vi "BonOMM-SAOMM.Test.vi"() -> ()   [LabVIEW 2011] (continued)
                        n1500 = case shown="False" w5027 {
                          frame False {
                            n1501 = One Button Dialog(message="ATTENTION!!\nLe télescope n'est pas en \nMODE ENTRAÎNEMENT SIDÉRAL.", button name ("OK")="OK" ("nom du bouton (\"OK\")")) -> ()  [unwired: 1 out]
                          }
                          frame True {
                          }
                        }
                      }
                    }
                  }
                }
                n1502 = case shown="True" w5001 {
                  frame False {
                  }
                  frame True {
                    n1503 = property on="GO" class="Bool (strict)"("Key Focus"=TRUE) -> ()  [unwired: 2 in, 2 out]
                  }
                }
              }
              event "SaveCoords": Value Change {
                n1504 = event-data() -> ()  [unwired: 1 in, 5 out]
                n1505 = flat-sequence {
                  tunnel: [w5039] -> w5035
                  tunnel: [w5038] -> w5034
                  tunnel: [w5037] -> w5033
                  tunnel: [w5036] -> w5032
                  tunnel: w5035 -> [w5045]
                  tunnel: w5034 -> [w5046]
                  tunnel: w5033 -> [w5047]
                  tunnel: w5032 -> [w5044]
                  frame #0 {
                    n1506 = local read "Epoch Tel"() -> (w5040:dbl)
                    n1507 = local read "DEC Tel"() -> (w5042:dbl)
                    n1508 = local read "RA Tel"() -> (w5041:dbl)
                    n1509 = local write "SaveCoords"(FALSE ("SaveCoords")) -> ()
                    n1510 = call "SaveCoords.vi"("Epoch Tel"=w5040, "DEC Tel"=w5042, "RA Tel"=w5041) -> ("Accepted?"=w5036:bool, "Epoch Out"=w5037:dbl, "DEC Out"=w5038:dbl, "RA Out"=w5039:dbl)  [unwired: 5 in]
                  }
                  frame #1 {
                    n1511 = case shown="True" w5044 {
                      tunnel: w5047 -> [_ w5051]
                      tunnel: w5046 -> [_ w5050]
                      tunnel: w5045 -> [_ w5049]
                      frame False {
                      }
                      frame True {
                        w5075 = "\t"
                        w5068 = "_"
                        w5062 = TRUE ("replace all? (F)")
                        w5061 = " "
                        w5060 = "0"
                        w5057 = i16 2 ("width (-)")
                        w5056 = i16 0 ("width (-)")
                        n1512 = call "time-sec-to-time-str-DEC.vi"("Numeric"=w5049) -> ("formatted-str"=w5072:string)
                        n1513 = call "time-sec-to-time-str-DEC.vi"("Numeric"=w5050) -> ("formatted-str"=w5073:string)
                        n1514 = Number To Fractional String(number=w5051, width (-)=i16 4, precision (6)=i16 2) -> (F-format string=w5074:string)  [unwired: 1 in]
                        n1515 = Get Date/Time String() -> (time string=w5071:string)  [unwired: 3 in, 1 out]
                        n1516 = local read "From library"() -> (w5052:bool)
                        n1517 = Concatenate Strings(w5071, w5075, w5072, w5075, w5073, w5075, w5074, "\r\n") -> (w5077:string)
                        n1518 = call "GetUTC.vi"() -> ("Day"=w5082:dbl, "Month"=w5081:dbl, "Year"=w5080:dbl)  [unwired: 6 out]
                        n1519 = case shown="True" w5052 {
                          tunnel: [FALSE FALSE] -> w5048
                          tunnel: w5072 -> [w5086 w5093]
                          tunnel: w5073 -> [w5085 w5094]
                          tunnel: w5074 -> [w5084 w5095]
                          tunnel: w5071 -> [w5083 w5092]
                          frame False {
                            w5088 = i16 0 items=["tel coords", "tel offset", "guidage"] ("options")
                            n1520 = local read "Obslib"() -> (w5089:string[][])
                            n1521 = Build Array(w5086, w5085, w5084, w5083) -> (w5090:string[])
                            n1522 = call "Coords to chart(new).vi"("DataLine"=w5090, "options"=w5088, "Tableau entrant"=w5089) -> ("historique"=w5091:string[][])
                            n1523 = local write "Obslib"(w5091) -> ()
                          }
                          frame True {
                            w5097 = i16 0 items=["tel coords", "tel offset", "guidage"] ("options")
                            n1524 = local read "Obslib"() -> (w5098:string[][])
                            n1525 = Build Array(w5093, w5094, w5095, w5092) -> (w5099:string[])
                            n1526 = call "Coords to chart(new).vi"("DataLine"=w5099, "options"=w5097, "Tableau entrant"=w5098) -> ("historique"=w5100:string[][])
                            n1527 = local write "Obslib"(w5100) -> ()
                          }
                        }
                        n1528 = Number To Fractional String(number=w5080, width (-)=i16 4, precision (6)=w5056) -> (F-format string=w5063:string)  [unwired: 1 in]
                        n1529 = Number To Fractional String(number=w5081, width (-)=w5057, precision (6)=w5056) -> (F-format string=w5058:string)  [unwired: 1 in]
                        n1530 = Number To Fractional String(number=w5082, width (-)=w5057, precision (6)=w5056) -> (F-format string=w5059:string)  [unwired: 1 in]
                        n1531 = Search and Replace String(replace all?=w5062, input string=w5058, search string=w5061, replace string=w5060) -> (result string=w5064:string)  [unwired: 4 in, 3 out]
                        n1532 = Search and Replace String(replace all?=w5062, input string=w5059, search string=w5061, replace string=w5060) -> (result string=w5065:string)  [unwired: 4 in, 3 out]
                        n1533 = local read "path_pointing"() -> (w5066:path)
                        n1534 = Concatenate Strings(w5063, w5068, w5064, w5068, w5065, ".pnt") -> (w5067:string)
                        n1535 = Build Path(base path=w5066, name or relative path=w5067) -> (appended path=w5070:path)
                        n1536 = local read "File I/O Error"() -> (w5079:errorcluster)
                        n1537 = Write to Text File(file (use dialog)=w5070, text=w5077, error in=w5079) -> (error out=w5078:errorcluster)  [unwired: 1 in, 2 out]
                        n1538 = local write "From library"(w5048) -> ()
                        n1539 = local write "File I/O Error"(w5078) -> ()
                      }
                    }
                  }
                }
              }
              event "NO RA clic-sim": Value Change; "N.O. A.D.": Mouse Down {
                n1540 = event-data() -> ()  [unwired: 1 in, 4 out]
                n1541 = local write "N.O. A.D."("") -> ()
                n1542 = local write "NO epoch"(2000.0 ("NO epoch")) -> ()
                "NO RA clic-sim" <- FALSE
              }
              event "N.O. Déc.": Mouse Down {
                n1543 = event-data() -> ()  [unwired: 1 in, 8 out]
                n1544 = local write "NO epoch"(2000.0 ("NO epoch")) -> ()
                n1545 = local write "N.O. Déc."("") -> ()
              }
              event "Zénith", "Écran", "Range": Value Change {
                n1546 = event-data() -> ()  [unwired: 1 in, 1 out]
                n1547 = local read "Mode Est"() -> (w5106:bool)
                n1548 = case shown="False" w5106 {
                  selector: w5106 -> [_ w5319]
                  frame False {
                    # "Track ON ou OFF"
                    n1549 = local read "STATL"() -> (w5111:bool[])
                    n1550 = Index Array(array=w5111, index=2 ("Index")) -> (element=w5110:bool)
                    n1551 = case shown="False" w5110 {
                      tunnel: "Range" -> [w5116 _]
                      tunnel: "Zénith" -> [w5115 _]
                      tunnel: "Écran" -> [w5114 _]
                      frame False {
                        w5113 = FALSE
                        w5119 = string[] ["RANGEMENT", "ZÉNITH", "ÉCRAN"]
                        w5124 = 0
                        n1552 = local read "TCS VRN"() -> (w5123:refnum<visa-resource-name>)
                        n1553 = control-ref of="TERMINAL"() -> (w5121:refnum<vi>)
                        n1554 = control-ref of="Indicateur d'état"() -> (w5122:refnum<vi>)
                        n1555 = Select(t=1, s=w5116, f=w5124) -> (s? t:f=w5132:i32)
                        n1556 = Select(t=2, s=w5115, f=w5124) -> (s? t:f=w5130:i32)
                        n1557 = Select(t=3, s=w5114, f=w5124) -> (s? t:f=w5131:i32)
                        n1558 = Compound Arithmetic op=ADD(w5132, w5130, w5131) -> (w5129:i32)
                        n1559 = local write "Zénith"(w5113) -> ()
                        n1560 = local write "Écran"(w5113) -> ()
                        n1561 = local write "Range"(w5113) -> ()
                        n1562 = Decrement(x=w5129) -> (x-1=w5120:i32)
                        n1563 = Index String Array(1:w5120, 2:w5119, 3:"Le télescope va se déplacer\nvers la position ") -> (0:w5128:string)
                        n1564 = Two Button Dialog(message=w5128, 1:"Annulez" ("Nom du bouton F (\"Annuler\")"), 2:"OK" ("Nom du bouton V (\"OK\")")) -> (T button?=w5136:bool)
                        n1565 = Index String Array(1:w5120, 2:w5119, 3:"Commande de déplacement : " ("string (\"\")")) -> (0:w5117:string)
                        n1566 = call "TERMINAL.vi"("Indicateur Refnum"=w5122, "Terminal Refnum"=w5121, "Indicateur d'état"=w5117) -> ()
                        n1567 = case shown="True" w5136 {
                          selector: w5136 -> [w5137 _]
                          tunnel: w5120 -> [_ w5141]
                          tunnel: w5116 -> [_ w5140]
                          tunnel: w5119 -> [_ w5139]
                          tunnel: w5123 -> [_ w5138]
                          frame False {
                            n1568 = local write "Zénith"(w5137) -> ()
                            n1569 = local write "Écran"(w5137) -> ()
                            n1570 = local write "Range"(w5137) -> ()
                          }
                          frame True {
                            n1571 = stacked-sequence {
                              seq-local: [w5143 _ _] -> [_ _ w5311]
                              tunnel: w5141 -> [w5144 w5172 _]
                              tunnel: w5140 -> [_ w5179 _]
                              tunnel: w5139 -> [_ w5178 _]
                              tunnel: w5138 -> [w5142 w5177 _]
                              frame #0 {
                                n1572 = disable-structure shown="Disabled" {
                                disable-tunnel: [w5146 _] -> w5143
                                disable-tunnel: w5142 -> [w5145 _]
                                frame Disabled {
                                n1573 = flat-sequence {
                                tunnel: [w5148] -> w5146
                                tunnel: w5145 -> [w5152]
                                tunnel: [w5150] -> w5147
                                tunnel: w5147 -> [w5155]
                                frame #0 {
                                n1574 = local read "Epoch Tel"() -> (w5149:dbl)
                                n1575 = Build Array(w5149) -> (w5148:dbl[])
                                }
                                frame #1 {
                                n1576 = local read "AnnéeRL"() -> (w5150:dbl)
                                n1577 = control-ref of="TCS actif"() -> (w5151:refnum<vi>)
                                n1578 = Build Array(w5150) -> (w5154:dbl[])
                                n1579 = call "EXCOM-CMD.vi"("VRN IN"=w5152, "Bool Refnum"=w5151, "Commande #"=22, "Args"=w5154) -> ()  [unwired: 9 in, 3 out]
                                }
                                frame #2 {
                                n1580 = while {
                                tunnel: [w5158] -> _
                                tunnel: w5155 -> [w5156]
                                i -> [w5165]
                                stop <- w5162 stop-if-true
                                # "Environ 1 jour ..."
                                n1581 = local read "Epoch Tel"() -> (w5161:dbl)
                                n1582 = Subtract(x=w5161, y=w5156) -> (x-y=w5160:dbl)
                                n1583 = Absolute Value(x=w5160) -> (abs(x)=w5159:dbl)
                                n1584 = Less Or Equal?(x=w5159, y=0.002) -> (x <= y?=w5158:bool)
                                n1585 = call "Max-iteration.vi"("i max"=500, "i act"=w5165, "Valeur entrante"=w5158) -> ("break ?"=w5162:bool)
                                n1586 = Wait (ms)(milliseconds to wait=u32 10) -> ()  [unwired: 1 out]
                                }
                                }
                                }
                                }
                                frame Enabled {
                                }
                                }
                                n1587 = disable-structure shown="Disabled" {
                                disable-tunnel: w5144 -> [w5166 _]
                                frame Disabled {
                                n1588 = case shown="2" w5166 {
                                frame 0, Default {
                                n1589 = property on="Range" class="Bool (strict)"("Blinking"=TRUE) -> ()  [unwired: 2 in, 2 out]
                                }
                                frame 1 {
                                n1590 = property on="Zénith" class="Bool (strict)"("Blinking"=TRUE) -> ()  [unwired: 2 in, 2 out]
                                }
                                frame 2 {
                                n1591 = property on="Écran" class="Bool (strict)"("Blinking"=TRUE) -> ()  [unwired: 2 in, 2 out]
                                }
                                }
                                }
                                frame Enabled {
                                }
                                }
                              }
                              frame #1 {
                                n1592 = case shown="2" w5172 {
                                selector: w5172 -> [w5282 w5286 w5290]
                                tunnel: [w5282 w5286 w5290] -> w5171
                                tunnel: [w5285 w5289 w5293] -> w5170
                                frame 0, Default {
                                n1593 = Build Array(4.0 ("element"), 10.0 ("element")) -> (w5285:dbl[])
                                }
                                frame 1 {
                                n1594 = Build Array(0.0 ("element"), 45.45556 ("element")) -> (w5289:dbl[])
                                }
                                frame 2 {
                                n1595 = Build Array(5.0 ("element"), 56.0 ("element")) -> (w5293:dbl[])
                                }
                                }
                                n1596 = property on="Position Z" class="DigNum (strict)" props=["Value"]() -> ()  [unwired: 2 in, 3 out]
                                n1597 = control-ref of="TCS actif"() -> (w5173:refnum<vi>)
                                n1598 = case shown="True" w5179 {
                                frame False {
                                }
                                frame True {
                                n1599 = Two Button Dialog(message="Ranger la sonde aussi?", 1:"Non" ("F button name (\"Cancel\")"), 2:"Oui" ("T button name (\"OK\")")) -> (T button?=w5294:bool)
                                n1600 = case shown="True" w5294 {
                                frame False {
                                }
                                frame True {
                                n1601 = local read "Table VRN"() -> (w5307:refnum<visa-resource-name>)
                                n1602 = local read "Table Error"() -> (w5299:errorcluster)
                                n1603 = local read "Rangement Y"() -> (w5303:dbl)
                                n1604 = local read "Rangement X"() -> (w5304:dbl)
                                n1605 = local read "Rangement Z"() -> (w5302:dbl)
                                n1606 = control-ref of="Table actif"() -> (w5308:refnum<vi>)
                                n1607 = call "Newmark-GotoAll.vi"("Table VRN IN"=w5307, "Bool Refnum"=w5308, "Notify?"=FALSE, "Error IN"=w5299, "Position X"=w5304, "Position Y"=w5303, "Position Z"=w5302) -> ("Table VRN OUT"=w5306:refnum<visa-resource-name>, "Error OUT"=w5298:errorcluster)  [unwired: 7 in]
                                n1608 = Unbundle By Name(w5298) -> ("status"=w5301:bool)
                                n1609 = local write "Table Error"(w5298) -> ()
                                n1610 = local write "Table VRN"(w5306) -> ()
                                n1611 = Not(x=w5301) -> (.not. x?=w5300:bool)
                                n1612 = case shown="True" w5300 {
                                frame False {
                                n1613 = One Button Dialog(message="ATTENTION!!\nLa commande RangeTable a échoué.\nVérifiez le contrôleur des tables.", button name ("OK")="OK" ("nom du bouton (\"OK\")")) -> ()  [unwired: 1 out]
                                }
                                frame True {
                                }
                                }
                                }
                                }
                                }
                                }
                                n1614 = call "EXCOM-CMD.vi"("VRN IN"=w5177, "Bool Refnum"=w5173, "Commande #"=36, "Args"=w5170) -> ("VRN OUT"=w5175:refnum<visa-resource-name>, "OK Done"=w5180:bool, "Error OUT"=w5174:errorcluster)  [unwired: 9 in]
                                n1615 = case shown="True" w5180 {
                                tunnel: w5178 -> [w5185 _]
                                tunnel: w5171 -> [w5184 w5208]
                                tunnel: w5175 -> [w5183 w5203]
                                tunnel: w5174 -> [w5182 w5202]
                                tunnel: w5173 -> [w5181 w5200]
                                frame False {
                                n1616 = Index String Array(1:w5184, 2:w5185, 3:"ATTENTION!!\nLa commande" ("chaîne (\"\")")) -> (0:w5189:string)
                                n1617 = Concatenate Strings(w5189, " a échoué.\nAnnulez la commande." ("chaîne")) -> (w5186:string)
                                n1618 = One Button Dialog(message=w5186, button name ("OK")="OK" ("nom du bouton (\"OK\")")) -> (true=w5190:bool)
                                n1619 = case shown="True" w5190 {
                                tunnel: w5183 -> [_ w5196]
                                tunnel: w5182 -> [_ w5195]
                                tunnel: w5181 -> [_ w5192]
                                frame False {
                                }
                                frame True {
                                n1620 = call "EXCOM-CMD.vi"("VRN IN"=w5196, "Bool Refnum"=w5192, "Commande #"=13, "Error IN"=w5195) -> ("OK Done"=w5193:bool)  [unwired: 9 in, 2 out]
                                n1621 = case shown="False" w5193 {
                                frame False {
                                n1622 = One Button Dialog(message="ATTENTION!!\nLa commande STOP a échoué.\nVérifiez TCS.", button name ("OK")="OK" ("nom du bouton (\"OK\")")) -> ()  [unwired: 1 out]
                                }
                                frame True {
                                n1623 = Wait (ms)(milliseconds to wait=u32 10 ("attente (ms)")) -> ()  [unwired: 1 out]
                                }
                                }
                                }
                                }
                                }
                                frame True {
                                # "Est-ce qu'ici on pourrait utiliser\nl'information déjà obtenue ?"
                                # "Drives ON ?"
                                n1624 = call "EXCOM-26.vi"("VRN IN"=w5203, "Bool Refnum"=w5200, "Error IN"=w5202) -> ("STATH"=w5205:bool[], "VRN OUT"=w5204:refnum<visa-resource-name>, "Error OUT"=w5201:errorcluster)  [unwired: 6 in, 4 out]
                                n1625 = Index Array(array=w5205, index=7 ("Index")) -> (element=w5206:bool)
                                n1626 = case shown="True" w5206 {
                                tunnel: w5208 -> [_ w5233]
                                tunnel: w5204 -> [w5213 w5232]
                                tunnel: w5201 -> [w5212 w5231]
                                tunnel: [w5209 w5230] -> _
                                tunnel: [w5211 w5229] -> _
                                tunnel: [w5210 w5228] -> _
                                tunnel: w5200 -> [_ w5227]
                                frame False {
                                n1627 = stacked-sequence {
                                tunnel: w5213 -> [_ w5221 _]
                                tunnel: w5212 -> [_ w5219 _]
                                tunnel: [_ w5218 _] -> w5209
                                tunnel: [_ w5217 _] -> w5211
                                tunnel: [_ w5216 _] -> w5210
                                frame #0 {
                                n1628 = One Button Dialog(message="ATTENTION!!\nLes moteurs ne sont pas allumés. ", button name ("OK")="OK" ("nom du bouton (\"OK\")")) -> ()  [unwired: 1 out]
                                }
                                frame #1 {
                                n1629 = call "EXCOM-CMD.vi"("VRN IN"=w5221, "Commande #"=13, "Error IN"=w5219) -> ("VRN OUT"=w5217:refnum<visa-resource-name>, "OK Done"=w5216:bool, "Error OUT"=w5218:errorcluster)  [unwired: 10 in]
                                n1630 = case shown="False" w5216 {
                                frame False {
                                n1631 = One Button Dialog(message="ATTENTION!!\nLa commande STOP a échoué.\nVérifiez TCS.", button name ("OK")="OK" ("nom du bouton (\"OK\")")) -> ()  [unwired: 1 out]
                                }
                                frame True {
                                n1632 = Wait (ms)(milliseconds to wait=u32 10 ("attente (ms)")) -> ()  [unwired: 1 out]
                                }
                                }
                                }
                                frame #2 {
                                w5225 = 0
                                w5226 = FALSE ("Blinking")
                                n1633 = property on="Zénith" class="Bool (strict)"("Disabled"=w5225) -> ()  [unwired: 2 in, 2 out]
                                n1634 = property on="Range" class="Bool (strict)"("Disabled"=w5225) -> ()  [unwired: 2 in, 2 out]
                                n1635 = property on="Écran" class="Bool (strict)"("Disabled"=w5225) -> ()  [unwired: 2 in, 2 out]
                                n1636 = property on="Zénith" class="Bool (strict)"("Blinking"=w5226) -> ()  [unwired: 2 in, 2 out]
                                n1637 = property on="Range" class="Bool (strict)"("Blinking"=w5226) -> ()  [unwired: 2 in, 2 out]
                                n1638 = property on="Écran" class="Bool (strict)"("Blinking"=w5226) -> ()  [unwired: 2 in, 2 out]
                                }
                                }
                                }
                                frame True {
                                n1639 = stacked-sequence {
                                tunnel: w5233 -> [w5248 _]
                                tunnel: w5232 -> [w5247 w5279]
                                tunnel: w5231 -> [_ w5277]
                                tunnel: [_ w5276] -> w5230
                                tunnel: [_ w5275] -> w5229
                                tunnel: [_ w5274] -> w5228
                                tunnel: w5227 -> [w5235 w5273]
                                frame #0 {
                                # "Est-ce qu'ici on pourrait utiliser\nl'information déjà obtenue ?"
                                n1640 = local read "dflt-EQX"() -> (w5234:dbl)
                                n1641 = call "EXCOM-25-EQ.vi"("VISA resource name"=w5247, "Bool Refnum"=w5235, "Display Equinox"=w5234) -> ("RA"=w5242:dbl, "DEC"=w5241:dbl, "Epoque"=w5236:dbl, "Temps Sidéral"=w5237:dbl)  [unwired: 2 in, 11 out]
                                n1642 = case shown="0" w5248 {
                                tunnel: w5237 -> [w5251 w5260 w5266 _]
                                tunnel: [w5250 w5260 w5262 w5272] -> w5244
                                tunnel: [36000.0 ("y") 163640.0 ("Nouvelle Déc.") 201600.0 ("Nouvelle Déc.") w5271] -> w5243
                                tunnel: w5242 -> [_ _ _ w5272]
                                tunnel: w5241 -> [_ _ _ w5271]
                                frame 0 {
                                n1643 = Subtract(x=w5251, y=14400.0) -> (x-y=w5252:dbl)
                                n1644 = Less Than 0?(x=w5252) -> (x < 0?=w5253:bool)
                                n1645 = case shown="True" w5253 {
                                tunnel: w5252 -> [w5255 w5257]
                                tunnel: [w5255 w5256] -> w5250
                                frame False {
                                }
                                frame True {
                                n1646 = Add(x=w5257, y=86400.0) -> (x+y=w5256:dbl)
                                }
                                }
                                }
                                frame 1 {
                                }
                                frame 2 {
                                n1647 = Subtract(x=w5266, y=18000.0 ("x")) -> (x-y=w5263:dbl)
                                n1648 = Less Than 0?(x=w5263) -> (x < 0?=w5264:bool)
                                n1649 = case shown="True" w5264 {
                                tunnel: w5263 -> [w5267 w5270]
                                tunnel: [w5267 w5269] -> w5262
                                frame False {
                                }
                                frame True {
                                n1650 = Add(x=w5270, y=86400.0) -> (x+y=w5269:dbl)
                                }
                                }
                                }
                                frame 3, Default {
                                }
                                }
                                n1651 = call "Object_properties.vi"("Target RA"=w5244, "Target DEC"=w5243, "Target Epoch"=w5236, "Sideral Time"=w5237) -> ("NO RA"=w5246:string, "NO DEC"=w5245:string, "NO Epoch"=w5240:dbl, "NO HA"=w5239:dbl, "NO AM"=w5238:dbl)  [unwired: 7 in]
                                n1652 = local write "NO epoch"(w5240) -> ()
                                n1653 = local write "NO AM"(w5238) -> ()
                                n1654 = local write "NO HA"(w5239) -> ()
                                n1655 = local write "N.O. Déc."(w5245) -> ()
                                n1656 = local write "N.O. A.D."(w5246) -> ()
                                }
                                frame #1 {
                                n1657 = call "EXCOM-CMD.vi"("VRN IN"=w5279, "Bool Refnum"=w5273, "Commande #"=12, "Error IN"=w5277) -> ("VRN OUT"=w5275:refnum<visa-resource-name>, "OK Done"=w5274:bool, "Error OUT"=w5276:errorcluster)  [unwired: 9 in]
                                n1658 = case shown="False" w5274 {
                                frame False {
                                n1659 = One Button Dialog(message="ATTENTION!!\nLa commande GO a échoué.\nRecommencez ou vérifiez TCS.", button name ("OK")="OK" ("nom du bouton (\"OK\")")) -> ()  [unwired: 1 out]
                                }
                                frame True {
                                }
                                }
                                }
                                }
                                }
                                }
                                }
                                }
                              }
                              frame #2 {
                                n1660 = disable-structure shown="Disabled" {
                                disable-tunnel: w5311 -> [w5312 _]
                                frame Disabled {
                                n1661 = control-ref of="TCS actif"() -> (w5313:refnum<vi>)
                                n1662 = local read "TCS VRN"() -> (w5314:refnum<visa-resource-name>)
                                n1663 = call "EXCOM-CMD.vi"("VRN IN"=w5314, "Bool Refnum"=w5313, "Commande #"=22, "Args"=w5312) -> ()  [unwired: 9 in, 3 out]
                                }
                                frame Enabled {
                                }
                                }
                              }
                            }
                          }
                        }
                      }
                      frame True {
                        w5316 = FALSE
                        n1664 = local write "Zénith"(w5316) -> ()
                        n1665 = local write "Écran"(w5316) -> ()
                        n1666 = local write "Range"(w5316) -> ()
                        n1667 = One Button Dialog(message="ATTENTION!!\nAssurez-vous que l'entraînement sidéral\nest éteint", button name ("OK")="OK" ("nom du bouton (\"OK\")")) -> ()  [unwired: 1 out]
                      }
                    }
                  }
                  frame True {
                    n1668 = local write "Zénith"(w5319) -> ()
                    n1669 = local write "Écran"(w5319) -> ()
                    n1670 = local write "Range"(w5319) -> ()
                    n1671 = One Button Dialog(message="ATTENTION!!\nLe télescope doit être en mode OUEST\npour atteindre cette position ", button name ("OK")="OK" ("nom du bouton (\"OK\")")) -> ()  [unwired: 1 out]
                  }
                }
              }
              event "Origine": Value Change {
                n1672 = event-data() -> ("NewVal"=w5322:bool)  [unwired: 1 in, 4 out]
                n1673 = case shown="True" w5322 {
                  selector: w5322 -> [_ w5323]
                  frame False {
                  }
                  frame True {
                    n1674 = flat-sequence {
                      tunnel: w5323 -> [_]
                      frame #0 {
                        w5325 = 0.0 ("Cible X")
                        n1675 = control-ref of="TERMINAL"() -> (w5329:refnum<vi>)
                        n1676 = control-ref of="Indicateur d'état"() -> (w5328:refnum<vi>)
                        n1677 = local write "Origine"(FALSE ("NeedOrigin")) -> ()
                        n1678 = local write "Cible X"(w5325) -> ()
                        n1679 = local write "Cible Y"(w5325) -> ()
                        n1680 = local write "Cible Z"(w5325) -> ()
                        n1681 = call "TERMINAL.vi"("Indicateur Refnum"=w5328, "Terminal Refnum"=w5329, "Indicateur d'état"="Commande d'origine des tables") -> ()
                        "Origine en cours..." <- TRUE ("Qsleep")
                      }
                      frame #1 {
                        n1682 = flat-sequence {
                          tunnel: [w5342] -> w5331
                          tunnel: [w5338] -> w5330
                          tunnel: w5331 -> [w5344]
                          tunnel: w5330 -> [w5343]
                          frame #0 {
                            # "Si F,F,F -> 0,0,0\nSi F,F,V -> 0,0,1000000"
                            # "Position X, Y, Z après l'initialisation"
                            # "Valeur de vitesse utilisées ..."
                            n1683 = local read "ActiveStages"() -> (w5336:string[])
                            n1684 = local read "Table VRN"() -> (w5332:refnum<visa-resource-name>)
                            n1685 = control-ref of="Exceptions"() -> (w5335:refnum<vi>)
                            n1686 = control-ref of="Table actif"() -> (w5337:refnum<vi>)
                            n1687 = local read "Table Error"() -> (w5339:errorcluster)
                            n1688 = control-ref of="Quit_Origine"() -> (w5334:refnum<vi>)
                            n1689 = call "Newmark-Home.vi"("Table VRN IN"=w5332, "Comm Active"=w5337, "Exceptions"=w5335, "StageTAGs"=w5336, "Velocities"=cluster{"Slow":dbl, "Fast":dbl, "Accel":dbl} {"Slow"=10.0, "Fast"=30000.0, "Accel"=60000.0}, "HomeReverse?"=bool[] [FALSE, FALSE, TRUE], "Error IN"=w5339, "Quit Orgine"=w5334, "EndValues"=i32[] [0, 0, 1000000]) -> ("Table VRN OUT"=w5342:refnum<visa-resource-name>, "Error OUT"=w5338:errorcluster)  [unwired: 5 in]
                          }
                          frame #1 {
                            n1690 = local write "Origine en cours..."(FALSE ("Origine en cours...")) -> ()
                            n1691 = local write "Table VRN"(w5344) -> ()
                            n1692 = local write "Table Error"(w5343) -> ()
                          }
                        }
                        n1693 = while {
                          stop <- w5349 continue-if-true
                          n1694 = Wait (ms)(milliseconds to wait=u32 333) -> ()  [unwired: 1 out]
                          n1695 = local read "enfoncé"() -> (w5346:bool)
                          n1696 = Not(x=w5346) -> (.not. x?=w5347:bool)
                          n1697 = local write "enfoncé"(w5347) -> ()
                          n1698 = local read "Origine en cours..."() -> (w5349:bool)
                        }
                      }
                      frame #2 {
                        w5350 = FALSE ("NeedOrigin")
                        n1699 = local write "NeedOrigin"(w5350) -> ()
                        n1700 = local write "enfoncé"(w5350) -> ()
                        n1701 = property on="Origine" class="Bool (strict)"("Blinking"=FALSE) -> ()  [unwired: 2 in, 2 out]
                      }
                    }
                  }
                }
              }
              event "Centre": Value Change {
                n1702 = event-data() -> ("NewVal"=w5353:bool)  [unwired: 1 in, 4 out]
                n1703 = local write "Centre"(FALSE ("Centre")) -> ()
                n1704 = case shown="True" w5353 {
                  frame False {
                  }
                  frame True {
                    w5354 = TRUE ("CorrectZ")
                    n1705 = control-ref of="TERMINAL"() -> (w5364:refnum<vi>)
                    n1706 = control-ref of="Indicateur d'état"() -> (w5365:refnum<vi>)
                    n1707 = local read "Reference X"() -> (w5357:dbl)
                    n1708 = local read "Reference Y"() -> (w5356:dbl)
                    n1709 = local read "Position Z"() -> (w5355:dbl)
                    n1710 = call "TERMINAL.vi"("Indicateur Refnum"=w5365, "Terminal Refnum"=w5364, "Indicateur d'état"="Commande de déplacement des tables vers le centre") -> ()
                    n1711 = local read "Table Error"() -> (w5359:errorcluster)
                    n1712 = local read "Table VRN"() -> (w5363:refnum<visa-resource-name>)
                    n1713 = control-ref of="Table actif"() -> (w5361:refnum<vi>)
                    n1714 = local write "CorrectXY"(w5354) -> ()
                    n1715 = local write "CurvCorrect"(w5354) -> ()
                    n1716 = call "Newmark-GotoAll.vi"("Table VRN IN"=w5363, "Bool Refnum"=w5361, "Notify?"=FALSE, "Error IN"=w5359, "Position X"=w5357, "Position Y"=w5356, "Position Z"=w5355) -> ("Table VRN OUT"=w5362:refnum<visa-resource-name>, "Error OUT"=w5358:errorcluster)  [unwired: 7 in]
                    n1717 = local write "Table VRN"(w5362) -> ()
                    n1718 = local write "Table Error"(w5358) -> ()
                    n1719 = local write "Cible X"(w5357) -> ()
                    n1720 = local write "Cible Y"(w5356) -> ()
                    n1721 = local write "Cible Z"(w5355) -> ()
                  }
                }
              }
              event "Alacible": Value Change {
                n1722 = event-data() -> ("NewVal"=w5368:bool)  [unwired: 1 in, 4 out]
                n1723 = case shown="True" w5368 {
                  frame False {
                  }
                  frame True {
                    w5369 = TRUE ("CorrectZ")
                    # "Calcul de la position\nde la sonde en pulse"
                    n1724 = property on="TableXYPos" class="XYGraph (strict)"("Active Cursor"=u32 0) -> ("Cursor.Cursor X"=w5394:dbl, "Cursor.Cursor Y"=w5393:dbl)  [unwired: 2 in, 2 out]
                    n1725 = local read "FieldAstrom"() -> (w5390:T4)
                    n1726 = call "xy2ad.vi"("Y (px)"=w5393, "X (px)"=w5394, "Astrometry"=w5390) -> ("DEC (°)"=w5391:dbl, "RA (°)"=w5392:dbl)  [unwired: 5 in, 2 out]
                    n1727 = local write "CorrectXY"(w5369) -> ()
                    n1728 = local write "CurvCorrect"(w5369) -> ()
                    n1729 = local read "TableAstrom"() -> (w5389:T4)
                    n1730 = call "ad2xy.vi"("DEC"=w5391, "RA"=w5392, "Astrometry"=w5389) -> ("Y"=w5372:dbl, "X"=w5374:dbl)  [unwired: 6 in, 1 out]
                    n1731 = Round To Nearest(number=w5374) -> (nearest integer value=w5373:dbl)
                    n1732 = Round To Nearest(number=w5372) -> (nearest integer value=w5371:dbl)
                    n1733 = Number To Fractional String(number=w5374, precision (6)=i16 0) -> (F-format string=w5379:string)  [unwired: 2 in]
                    n1734 = Number To Fractional String(number=w5372, precision (6)=i16 0) -> (F-format string=w5378:string)  [unwired: 2 in]
                    n1735 = local read "Position Z"() -> (w5370:dbl)
                    n1736 = Concatenate Strings("Commande de déplacement des tables vers la cible [" ("Indicateur d'état"), w5379, "," ("Indicateur d'état"), w5378, "]" ("Indicateur d'état")) -> (w5375:string)
                    n1737 = control-ref of="TERMINAL"() -> (w5397:refnum<vi>)
                    n1738 = control-ref of="Indicateur d'état"() -> (w5396:refnum<vi>)
                    n1739 = local write "Cible X"(w5373) -> ()
                    n1740 = local write "Cible Y"(w5371) -> ()
                    n1741 = local write "Cible Z"(w5370) -> ()
                    n1742 = call "TERMINAL.vi"("Indicateur Refnum"=w5396, "Terminal Refnum"=w5397, "Indicateur d'état"=w5375) -> ()
                    n1743 = local read "Table VRN"() -> (w5388:refnum<visa-resource-name>)
                    n1744 = local read "Table Error"() -> (w5386:errorcluster)
                    n1745 = control-ref of="Table actif"() -> (w5383:refnum<vi>)
                    n1746 = call "Newmark-GotoAll.vi"("Table VRN IN"=w5388, "Bool Refnum"=w5383, "Notify?"=FALSE, "Error IN"=w5386, "Position X"=w5373, "Position Y"=w5371, "Position Z"=w5370) -> ("Table VRN OUT"=w5387:refnum<visa-resource-name>, "Error OUT"=w5385:errorcluster)  [unwired: 7 in]
                    n1747 = local write "Table VRN"(w5387) -> ()
                    n1748 = local write "Table Error"(w5385) -> ()
                  }
                }
                n1749 = local write "Alacible"(FALSE ("Alacible")) -> ()
              }
              event "Calibration": Value Change {
                w5398 = TRUE ("CorrectZ")
                n1750 = event-data() -> ("NewVal"=w5400:bool)  [unwired: 1 in, 4 out]
                n1751 = local write "CorrectXY"(w5398) -> ()
                n1752 = local write "CurvCorrect"(w5398) -> ()
                n1753 = local write "Calibration"(FALSE ("Calibration")) -> ()
                n1754 = case shown="True" w5400 {
                  frame False {
                  }
                  frame True {
                    n1755 = control-ref of="TERMINAL"() -> (w5410:refnum<vi>)
                    n1756 = control-ref of="Indicateur d'état"() -> (w5411:refnum<vi>)
                    n1757 = call "TERMINAL.vi"("Indicateur Refnum"=w5411, "Terminal Refnum"=w5410, "Indicateur d'état"="Commande de déplacement des tables vers la position de calibration.") -> ()
                    n1758 = local read "Table VRN"() -> (w5409:refnum<visa-resource-name>)
                    n1759 = local read "Table Error"() -> (w5407:errorcluster)
                    n1760 = local read "Position Z"() -> (w5401:dbl)
                    n1761 = control-ref of="Table actif"() -> (w5404:refnum<vi>)
                    n1762 = call "Newmark-GotoAll.vi"("Table VRN IN"=w5409, "Bool Refnum"=w5404, "Notify?"=FALSE, "Error IN"=w5407, "Position X"="Calibration X", "Position Y"="Calibration Y", "Position Z"=w5401) -> ("Table VRN OUT"=w5408:refnum<visa-resource-name>, "Error OUT"=w5406:errorcluster)  [unwired: 7 in]
                    n1763 = local write "Table VRN"(w5408) -> ()
                    n1764 = local write "Table Error"(w5406) -> ()
                    n1765 = local write "Cible X"("Calibration X") -> ()
                    n1766 = local write "Cible Y"("Calibration Y") -> ()
                    n1767 = local write "Cible Z"(w5401) -> ()
                  }
                }
              }
              event "RangeTable": Value Change {
                n1768 = event-data() -> ("NewVal"=w5414:bool)  [unwired: 1 in, 4 out]
                n1769 = local write "RangeTable"(FALSE ("RangeTable")) -> ()
                n1770 = case shown="True" w5414 {
                  frame False {
                  }
                  frame True {
                    n1771 = local read "Table VRN"() -> (w5423:refnum<visa-resource-name>)
                    n1772 = local read "Table Error"() -> (w5421:errorcluster)
                    n1773 = control-ref of="TERMINAL"() -> (w5426:refnum<vi>)
                    n1774 = control-ref of="Indicateur d'état"() -> (w5425:refnum<vi>)
                    n1775 = control-ref of="Table actif"() -> (w5418:refnum<vi>)
                    n1776 = call "Newmark-GotoAll.vi"("Table VRN IN"=w5423, "Bool Refnum"=w5418, "Notify?"=FALSE, "Error IN"=w5421, "Position X"="Rangement Y", "Position Y"="Rangement X", "Position Z"="Rangement Z") -> ("Table VRN OUT"=w5422:refnum<visa-resource-name>, "Error OUT"=w5420:errorcluster)  [unwired: 7 in]
                    n1777 = call "TERMINAL.vi"("Indicateur Refnum"=w5425, "Terminal Refnum"=w5426, "Indicateur d'état"="Commande de rangement des tables") -> ()
                    n1778 = local write "Table VRN"(w5422) -> ()
                    n1779 = local write "Table Error"(w5420) -> ()
                    n1780 = local write "Cible X"("Rangement Y") -> ()
                    n1781 = local write "Cible Y"("Rangement X") -> ()
                    n1782 = local write "Cible Z"("Rangement Z") -> ()
                  }
                }
              }
              event "GO": Value Change {
                n1783 = event-data() -> ()  [unwired: 1 in, 5 out]
                n1784 = flat-sequence {
                  frame #0 {
                    n1785 = control-ref of="TERMINAL"() -> (w5429:refnum<vi>)
                    n1786 = control-ref of="Indicateur d'état"() -> (w5428:refnum<vi>)
                    n1787 = local write "GO"(FALSE) -> ()
                    n1788 = call "TERMINAL.vi"("Indicateur Refnum"=w5428, "Terminal Refnum"=w5429, "Indicateur d'état"="Commande de déplacement du télescope") -> ()
                  }
                  frame #1 {
                    n1789 = local read "STATH"() -> (w5431:bool[])
                    n1790 = Index Array(array=w5431, index=7 ("Index")) -> (element=w5432:bool)
                    n1791 = case shown="True" w5432 {
                      frame False {
                        w5434 = u32 0
                        # "Est-ce qu'on ne veut pas envoyez un stop à ce moment là ?"
                        n1792 = local read "FIFO d'erreur"() -> (w5436:T7)
                        n1793 = Bundle("TCS", w5434, w5434, "ATTENTION!!\nLes moteurs ne sont pas allumés.") -> (w5437:cluster{string, u32, u32, string})  [unwired: 1 in]
                        n1794 = Build Array (concatenate)(w5436, w5437) -> (w5435:T7)
                        n1795 = local write "FIFO d'erreur"(w5435) -> ()
                      }
                      frame True {
                        n1796 = control-ref of="TCS actif"() -> (w5440:refnum<vi>)
                        n1797 = local read "TCS VRN"() -> (w5441:refnum<visa-resource-name>)
                        n1798 = call "EXCOM-CMD.vi"("VRN IN"=w5441, "Bool Refnum"=w5440, "Commande #"=12) -> ("VRN OUT"=w5444:refnum<visa-resource-name>, "OK Done"=w5443:bool, "Error OUT"=w5442:errorcluster)  [unwired: 10 in]
                        n1799 = local write "TCS VRN"(w5444) -> ()
                        n1800 = local write "TCS Error"(w5442) -> ()
                        n1801 = case shown="True" w5443 {
                          selector: w5443 -> [_ w5448]
                          frame False {
                            n1802 = One Button Dialog(message="ATTENTION!!\nProblème de communication\navec TCS-Ctrl", button name ("OK")="OK" ("nom du bouton (\"OK\")")) -> ()  [unwired: 1 out]
                          }
                          frame True {
                            "Déplacement usager" <- w5448
                          }
                        }
                      }
                    }
                  }
                }
              }
              event "Synctel": Value Change {
                n1803 = event-data() -> ()  [unwired: 1 in, 5 out]
                n1804 = local read "Mode Est"() -> (w5449:bool)
                n1805 = case shown="False" w5449 {
                  frame False {
                    n1806 = flat-sequence {
                      frame #0 {
                        n1807 = local write "Synctel"(FALSE) -> ()
                      }
                      frame #1 {
                        w5454 = ", " ("F button name (\"Cancel\")")
                        n1808 = local read "NO epoch"() -> (w5460:dbl)
                        n1809 = local read "N.O. A.D."() -> (w5456:string)
                        n1810 = local read "N.O. Déc."() -> (w5453:string)
                        n1811 = Number To Fractional String(number=w5460, width (-)=i16 6, precision (6)=i16 2) -> (F-format string=w5452:string)  [unwired: 1 in]
                        n1812 = Concatenate Strings("êtes vous certain de vouloir synchroniser \nles coordonnées de TCS sur :\nR.A. : " ("string"), w5456, "\nDEC : ", w5453, "\nEPOCH : ", w5452) -> (w5464:string)
                        n1813 = control-ref of="TERMINAL"() -> (w5458:refnum<vi>)
                        n1814 = control-ref of="Indicateur d'état"() -> (w5457:refnum<vi>)
                        n1815 = Concatenate Strings("Synchronisation sur : " ("Indicateur d'état"), w5456, w5454, w5453, w5454, w5452) -> (w5451:string)
                        n1816 = Two Button Dialog(message=w5464, 1:"NON" ("F button name (\"Cancel\")"), 2:"OUI" ("T button name (\"OK\")")) -> (T button?=w5466:bool)
                        n1817 = call "TERMINAL.vi"("Indicateur Refnum"=w5457, "Terminal Refnum"=w5458, "Indicateur d'état"=w5451) -> ()
                        n1818 = case shown="True" w5466 {
                          tunnel: w5453 -> [_ w5480]
                          tunnel: w5456 -> [_ w5479]
                          frame False {
                          }
                          frame True {
                            # "Initialise RA et DEC\naux valeurs de Starry Night"
                            n1819 = local read "NO epoch"() -> (w5476:dbl)
                            n1820 = call "time-str-to-time-dbl-RA.vi"("Chaîne"=w5479) -> ("TCS_coords"=w5474:dbl)
                            n1821 = call "time-str-to-time-dbl-DEC.vi"("Chaîne"=w5480) -> ("TCS_coords"=w5475:dbl)
                            n1822 = control-ref of="TCS actif"() -> (w5469:refnum<vi>)
                            n1823 = local read "TCS VRN"() -> (w5477:refnum<visa-resource-name>)
                            n1824 = Build Array(w5474, w5475, w5476) -> (w5473:dbl[])
                            n1825 = call "EXCOM-CMD.vi"("VRN IN"=w5477, "Bool Refnum"=w5469, "Commande #"=3 ("NombredArguments"), "Args"=w5473) -> ("VRN OUT"=w5470:refnum<visa-resource-name>, "OK Done"=w5471:bool, "Error OUT"=w5472:errorcluster)  [unwired: 9 in]
                            n1826 = local write "TCS Error"(w5472) -> ()
                            n1827 = local write "TCS VRN"(w5470) -> ()
                            n1828 = case shown="False" w5471 {
                              frame False {
                                n1829 = One Button Dialog(message="ATTENTION!!\nLa commande SyncTEL a échoué.\nVérifiez TCS.", button name ("OK")="OK" ("nom du bouton (\"OK\")")) -> ()  [unwired: 1 out]
                              }
                              frame True {
                              }
                            }
                          }
                        }
                      }
                      frame #2 {
                        n1830 = control-ref of="TCS actif"() -> (w5483:refnum<vi>)
                        n1831 = local read "TCS VRN"() -> (w5485:refnum<visa-resource-name>)
                        n1832 = local read "TCS Error"() -> (w5484:errorcluster)
                        n1833 = call "EXCOM-CMD.vi"("VRN IN"=w5485, "Bool Refnum"=w5483, "Commande #"=13 ("NombredArguments"), "Error IN"=w5484) -> ("VRN OUT"=w5487:refnum<visa-resource-name>, "Error OUT"=w5486:errorcluster)  [unwired: 9 in, 1 out]
                        n1834 = local write "TCS VRN"(w5487) -> ()
                        n1835 = local write "TCS Error"(w5486) -> ()
                      }
                    }
                  }
                  frame True {
                    n1836 = One Button Dialog(message="Impossible de synchroniser les coordonnées en mode inversé.", button name ("OK")="Ok") -> ()  [unwired: 1 out]
                  }
                }
              }
              event "RotationTCS": Value Change {
                n1837 = event-data() -> ()  [unwired: 1 in, 5 out]
              }
              event "ModifRotation": Value Change {
                n1838 = event-data() -> ()  [unwired: 1 in, 5 out]
                n1839 = case shown="True" "ModifRotation" {
                  frame False {
                  }
                  frame True {
                    n1840 = local read "RotationTCS"() -> (w5499:dbl)
                    n1841 = control-ref of="TCS actif"() -> (w5492:refnum<vi>)
                    n1842 = local read "TCS VRN"() -> (w5496:refnum<visa-resource-name>)
                    n1843 = call "Set rotation.vi"("Rot.In"=w5499) -> ("DONE"=w5498:bool, "Rot.Out"=w5497:dbl)
                    n1844 = case shown="True" w5498 {
                      selector: w5498 -> [w5500 _]
                      tunnel: w5497 -> [_ w5503]
                      tunnel: w5496 -> [_ w5507]
                      tunnel: w5492 -> [_ w5506]
                      frame False {
                        n1845 = local write "ModifRotation"(w5500) -> ()
                      }
                      frame True {
                        n1846 = In Range and Coerce(upper limit=180.0, x=w5503, lower limit=0.0 ("upper limit")) -> (coerced(x)=w5501:dbl, In Range?=w5502:bool)
                        n1847 = case shown="True" w5502 {
                          tunnel: w5507 -> [_ w5512]
                          tunnel: w5506 -> [_ w5511]
                          tunnel: w5501 -> [_ w5509]
                          frame False {
                            n1848 = One Button Dialog(message="Les valeurs envoyées doivent être comprises entre 0° et 180°") -> ()  [unwired: 1 in, 1 out]
                          }
                          frame True {
                            # "Bug TCS"
                            n1849 = expression code="90-x"(w5509) -> (w5510:dbl)
                            n1850 = stacked-sequence {
                              tunnel: w5510 -> [_ w5518 _]
                              tunnel: w5512 -> [_ w5522 _]
                              tunnel: w5511 -> [_ w5516 _]
                              frame #0 {
                                w5514 = 2
                                w5513 = 2
                                # "Attendre 0.5 sec afin que la boucle de surveillance se termine"
                                n1851 = property on="ModifRotation" class="Bool (strict)"("Blinking"=TRUE) -> ()  [unwired: 2 in, 2 out]
                                n1852 = property on="GO" class="Bool (strict)"("Disabled"=w5513) -> ()  [unwired: 2 in, 2 out]
                                n1853 = property on="ModCoor" class="Bool (strict)"("Disabled"=w5513) -> ()  [unwired: 2 in, 2 out]
                                n1854 = property on="Synctel" class="Bool (strict)"("Disabled"=w5513) -> ()  [unwired: 2 in, 2 out]
                                n1855 = property on="Offset OK" class="Bool (strict)"("Disabled"=w5513) -> ()  [unwired: 2 in, 2 out]
                                n1856 = property on="Zénith" class="Bool (strict)"("Disabled"=w5514) -> ()  [unwired: 2 in, 2 out]
                                n1857 = property on="Écran" class="Bool (strict)"("Disabled"=w5514) -> ()  [unwired: 2 in, 2 out]
                                n1858 = property on="ModifFoyer" class="Bool (strict)"("Disabled"=w5514) -> ()  [unwired: 2 in, 2 out]
                                n1859 = property on="Range" class="Bool (strict)"("Disabled"=w5514) -> ()  [unwired: 2 in, 2 out]
                                n1860 = property on="ModifDome" class="Bool (strict)"("Disabled"=w5514) -> ()  [unwired: 2 in, 2 out]
                                n1861 = property on="Coupole-Tél" class="Bool (strict)"("Disabled"=w5514) -> ()  [unwired: 2 in, 2 out]
                              }
                              frame #1 {
                                # "Changement de la \nposition du rotateur."
                                n1862 = Build Array(w5518) -> (w5519:dbl[])
                                n1863 = call "EXCOM-CMD.vi"("VRN IN"=w5522, "Bool Refnum"=w5516, "Commande #"=4, "Args"=w5519) -> ("VRN OUT"=w5520:refnum<visa-resource-name>, "OK Done"=w5523:bool, "Error OUT"=w5517:errorcluster)  [unwired: 9 in]
                                n1864 = case shown="True" w5523 {
                                selector: w5523 -> [w5526 _]
                                tunnel: w5520 -> [w5524 w5540]
                                tunnel: w5517 -> [w5525 w5539]
                                tunnel: [w5525 w5538] -> _
                                tunnel: [w5524 w5537] -> _
                                tunnel: [w5526 w5536] -> _
                                tunnel: w5516 -> [_ w5535]
                                frame False {
                                w5527 = 4
                                n1865 = local read "CmdPending"() -> (w5528:bool)
                                n1866 = local read "FIFO d'erreur"() -> (w5532:T7)
                                n1867 = case shown="True" w5528 {
                                tunnel: w5527 -> [_ w5534]
                                frame False {
                                }
                                frame True {
                                n1868 = local write "Error Code"(w5534) -> ()
                                }
                                }
                                n1869 = Bundle("ETCS", w5527, w5527, "ATTENTION !!!\nLa commande MODIF-ROTATION a échoué.\nRecommencez ou vérifiez TCS.") -> (w5531:cluster{string, i32, i32, string})  [unwired: 1 in]
                                n1870 = Build Array (concatenate)(w5532, w5531) -> (w5533:T7)
                                n1871 = local write "FIFO d'erreur"(w5533) -> ()
                                }
                                frame True {
                                n1872 = stacked-sequence {
                                tunnel: w5540 -> [_ w5550]
                                tunnel: w5539 -> [_ w5549]
                                tunnel: [_ w5546] -> w5538
                                tunnel: [_ w5545] -> w5537
                                tunnel: [_ w5544] -> w5536
                                tunnel: w5535 -> [_ w5542]
                                frame #0 {
                                # "Devrait probablement vérifier l'état du flag à la place ..."
                                # "attendre 600ms que la commande GO soit acceptée par TCS"
                                n1873 = Wait (ms)(milliseconds to wait=u32 600 ("attente (ms)")) -> ()  [unwired: 1 out]
                                }
                                frame #1 {
                                n1874 = Tick Count (ms)() -> (millisecond timer value=w5552:u32)
                                n1875 = while {
                                tunnel: w5552 -> [w5566]
                                tunnel: [w5563] -> w5551
                                tunnel: w5550 -> [w5558]
                                tunnel: w5549 -> [w5557]
                                tunnel: [w5556] -> w5548
                                tunnel: [w5555] -> w5547
                                tunnel: [w5554] -> w5543
                                tunnel: w5542 -> [w5553]
                                stop <- w5565 stop-if-true
                                # "Max 90 secondes"
                                # "Bit 1 = slew ON ou OFF"
                                n1876 = Tick Count (ms)() -> (millisecond timer value=w5567:u32)
                                n1877 = call "EXCOM-26.vi"("VRN IN"=w5558, "Bool Refnum"=w5553, "Error IN"=w5557) -> ("VRN OUT"=w5556:refnum<visa-resource-name>, "OK Done"=w5554:bool, "STATEX"=w5559:bool[], "Error OUT"=w5555:errorcluster)  [unwired: 6 in, 3 out]
                                n1878 = Wait Until Next ms Multiple(millisecond multiple=u32 500 ("n millisecondes")) -> ()  [unwired: 1 out]
                                n1879 = Subtract(x=w5567, y=w5566) -> (x-y=w5568:u32)
                                n1880 = Greater?(x=w5568, y=u32 90000) -> (0:w5563:bool)
                                n1881 = Index Array(array=w5559, index=1 ("Index")) -> (element=w5560:bool)
                                n1882 = Not(x=w5560) -> (.not. x?=w5562:bool)
                                n1883 = Or(x=w5562, y=w5563) -> (x .or. y?=w5565:bool)
                                }
                                n1884 = case shown="True" w5551 {
                                tunnel: w5548 -> [w5571 w5578]
                                tunnel: w5547 -> [w5570 w5577]
                                tunnel: [w5570 w5576] -> w5546
                                tunnel: [w5571 w5575] -> w5545
                                tunnel: [w5572 w5574] -> w5544
                                tunnel: w5543 -> [w5572 _]
                                tunnel: w5542 -> [_ w5573]
                                frame False {
                                }
                                frame True {
                                w5585 = 4
                                n1885 = local read "CmdPending"() -> (w5579:bool)
                                n1886 = case shown="True" w5579 {
                                tunnel: w5585 -> [_ w5587]
                                frame False {
                                }
                                frame True {
                                n1887 = local write "Error Code"(w5587) -> ()
                                }
                                }
                                n1888 = call "EXCOM-CMD.vi"("VRN IN"=w5578, "Bool Refnum"=w5573, "Commande #"=13 ("NombredArguments"), "Error IN"=w5577) -> ("VRN OUT"=w5575:refnum<visa-resource-name>, "OK Done"=w5574:bool, "Error OUT"=w5576:errorcluster)  [unwired: 9 in]
                                n1889 = local read "FIFO d'erreur"() -> (w5583:T7)
                                n1890 = Bundle("ETCS", w5585, w5585, "Le rotateur ne semble pas avoir atteint sa position") -> (w5582:cluster{string, i32, i32, string})  [unwired: 1 in]
                                n1891 = Build Array (concatenate)(w5583, w5582) -> (w5584:T7)
                                n1892 = local write "FIFO d'erreur"(w5584) -> ()
                                n1893 = case shown="False" w5574 {
                                frame False {
                                w5589 = 128
